vi "oef5.vi"() -> ()   [LabVIEW 2021]
panel:
  in  "sinus 2":dbl(knob) scale=0.0..10000.0
  in  "sinus 1":dbl(knob) scale=0.0..10000.0
  in  "stop":bool
  out "Waveform Graph":dynamicdata(graph)
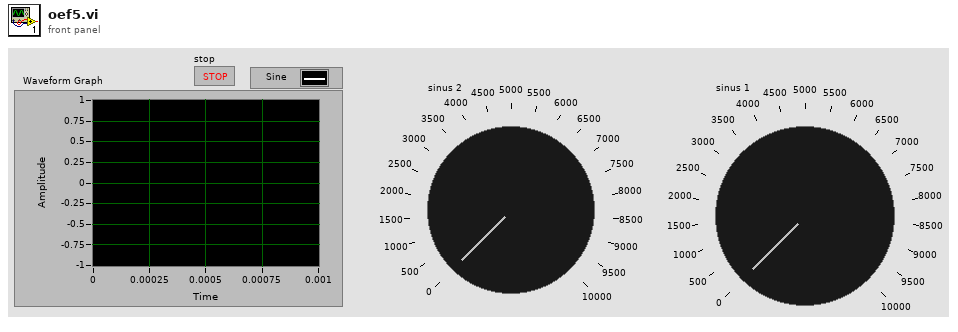
[diagram p1: front panel]
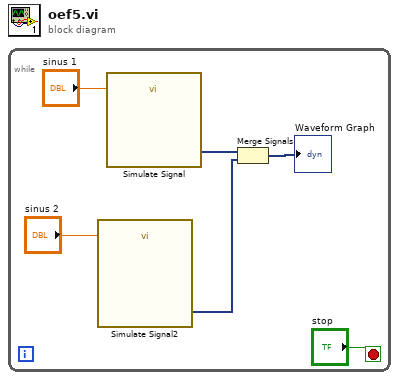
[diagram p0: block diagram]
diagram:
  n1 = while {
    stop <- "stop" stop-if-true
    n2 = call "Simulate Signal2"("Frequency"="sinus 2") -> ("Sine"=w1:dynamicdata)  [unwired: 13 in, 1 out]
    n3 = call "Simulate Signal"("Frequency"="sinus 1") -> ("Sine"=w6:dynamicdata)  [unwired: 13 in, 1 out]
    n4 = Merge Signals(w6, w1) -> (→"Waveform Graph":dynamicdata)
  }
